vi "test_fpga_se_main.vi"() -> ()   [LabVIEW 2016]
uses:
  <vilib>/Platform/TimedLoop/XDataNode/timing_clust.ctl
  <vilib>/Platform/TimedLoop/XDataNode/nitl_modes.ctl
  <vilib>/Platform/TimedLoop/XDataNode/wakeup.ctl
  <vilib>/rvi/Emulation/niFpgaSctlEmulationGetInTimedLoop.vi
  <vilib>/rvi/Emulation/niFpgaEmulationReportErrorSimple.vi
  <vilib>/rvi/Emulation/niFpgaGetClockAttributes.vi
  <vilib>/rvi/Emulation/niFpgaCriticalErrorInLSC.vi
  <vilib>/Platform/TimedLoop/XDataNode/XDataNode.xnode
  <vilib>/Platform/TimedLoop/XDataNode/XDNodeRunTimeDep.lvlib
panel:
  out "debug":cluster{"blanking":u32, "pixelEvent":bool}
  out "se.o.position":T1 {"outputInt"."x" format="%.16g"; "outputInt"."y" format="%.16g"}
  out "blankingOff":bool
  in  "scanClocks":T2={"se.mot.p.clocks"={"moveToDecFactor"=0, "moveToWaveSize"=0, "se.mot.p.invDec"=0.0}, "se.p.clocks"={"outputRate"=0, "fastDecFactor"=0, "outWaveSizeFast"=0, "pplUpsampling"=0, "numLines"=0, "se.p.fastInvDec"=0.0, "se.p.slowUpStep"=0.0, "se.p.outWaveSizeSlow"=0, "blankingMax"=0, "se.p.fastBlanking"={"startFwd"=0, "endFwd"=0, "startBwd"=0, "endBwd"=0, "disableBlanking"=FALSE, "useCoarseCounter"=TRUE}}}
  out "indices":T3
  in  "outputParams":T4
  out "se.mot.s.running":bool
  out "outputNorm":T5
  out "clocksOut":T6
  in  "se.p.modes":T7
  in  "se.mot.p.target":cluster{"x":fxp<+/-,16,1>, "y":fxp<+/-,16,1>}
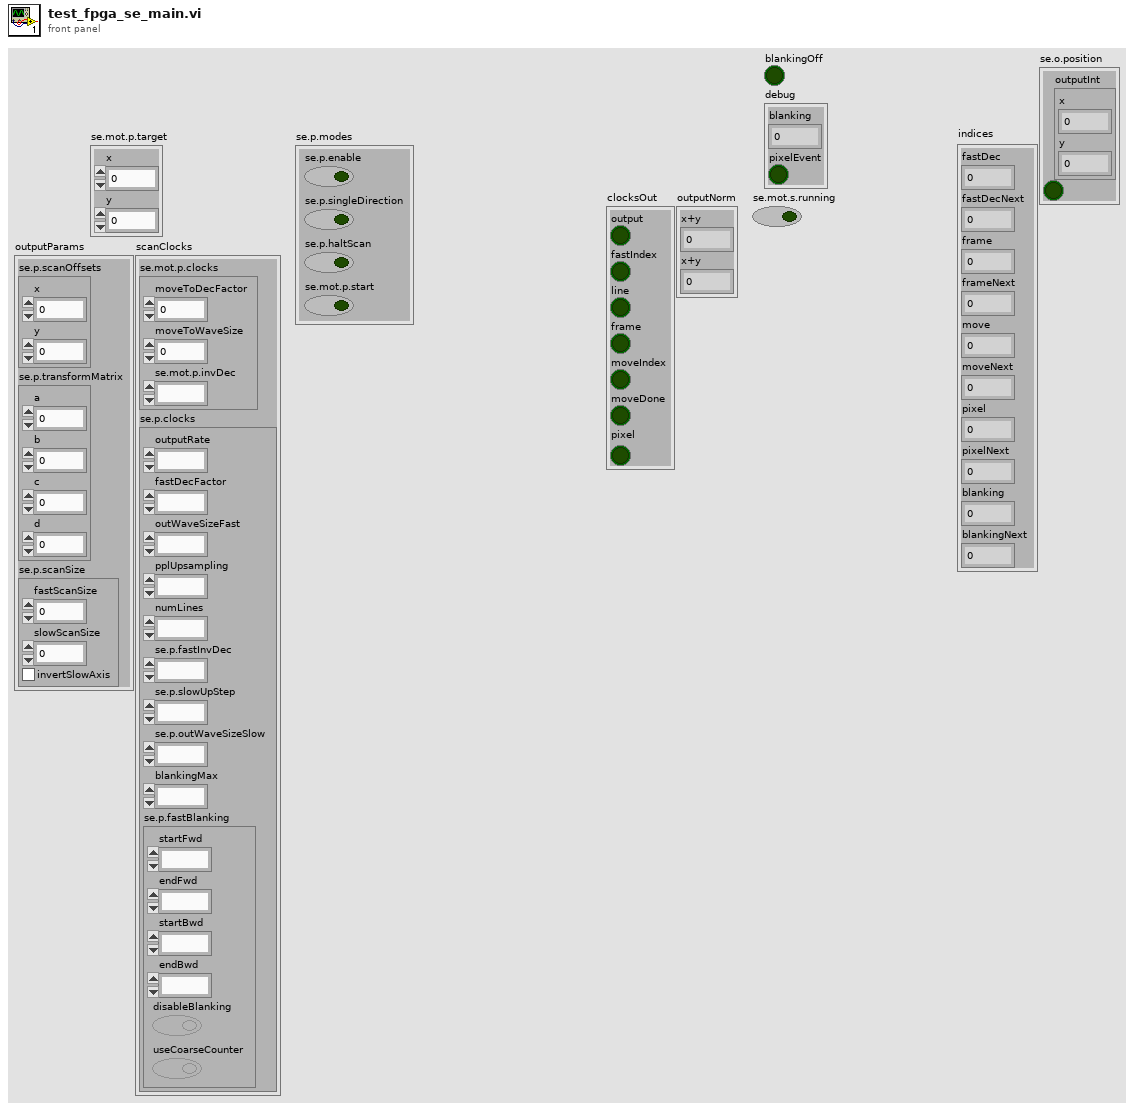
[diagram p1: front panel]
types:
  T1 = cluster{"outputInt":cluster{"y":fxp<+/-,16,1>, "y":fxp<+/-,16,1>}, bool}
  T2 = cluster{"se.mot.p.clocks":cluster{"moveToDecFactor":u16, "moveToWaveSize":u16, "se.mot.p.invDec":fxp<+,16,0>}, "se.p.clocks":cluster{"outputRate":u16, "fastDecFactor":u16, "outWaveSizeFast":u16, "pplUpsampling":u16, "numLines":u16, "se.p.fastInvDec":fxp<+,22,0>, "se.p.slowUpStep":fxp<+,28,0>, "se.p.outWaveSizeSlow":u16, "blankingMax":u32, "se.p.fastBlanking":cluster{"startFwd":u32, "endFwd":u32, "startBwd":u32, "endBwd":u32, "disableBlanking":bool, "useCoarseCounter":bool}}}
  T3 = cluster{"fastDec":u16, "fastDecNext":u16, "frame":u16, "frameNext":u16, "move":u16, "moveNext":u16, "pixel":u16, "pixelNext":u16, "blanking":u32, "blankingNext":u32}
  T4 = cluster{"se.p.scanOffsets":cluster{"x":fxp<+/-,16,1>, "y":fxp<+/-,16,1>}, "se.p.transformMatrix":cluster{"a":fxp<+/-,18,2>, "b":fxp<+/-,18,2>, "c":fxp<+/-,18,2>, "d":fxp<+/-,18,2>}, "se.p.scanSize":cluster{"fastScanSize":fxp<+,17,1>, "slowScanSize":fxp<+,17,1>, "invertSlowAxis":bool}}
  T5 = cluster{"x+y":fxp<+/-,18,2>, "x+y":fxp<+/-,18,2>}
  T6 = cluster{"output":bool, "fastIndex":bool, "line":bool, "frame":bool, "moveIndex":bool, "moveDone":bool, "pixel":bool}
  T7 = cluster{"se.p.enable":bool, "se.p.singleDirection":bool, "se.p.haltScan":bool, "se.mot.p.start":bool}
  T8 = typedef "XDNodeRunTimeDep.lvlib/timing_clust.ctl" = cluster{"Expected End [f-1]":u64, "Actual End [f-1]":u64, "Finished Late? [f-1]":bool, "Expected End [i-1]":u64, "Actual End [i-1]":u64, "Finished Late? [i-1]":bool, "Expected Start [i]":u64, "Actual Start [i]":u64, "Expected Start [f]":u64, "Actual Start [f]":u64, "Source Name":string, "Structure Name":string, "Period":i64, "Deadline":i64, "Offset":i64, "Start":i64, "Priority":i32, "Timeout":i32, "Mode":T9, "Wakeup Reason":T10, "Error":errorcluster, "Source Type":string, "Secondary Source Type":string, "Global End Time":u64, "Global Start Time":u64, "Frame Duration":u64, "Iteration Duration":u64, "Assigned CPU":i32, "I/O Scan Engine Mode":u32}
  T9 = typedef "XDNodeRunTimeDep.lvlib/nitl_modes.ctl" = enum32{"No Change", "Process missed periods, maintain original phase", "Discard missed periods, maintain original phase", "Process missed periods, ignore original phase", "Discard missed periods, ignore original phase"}
  T10 = typedef "XDNodeRunTimeDep.lvlib/wakeup.ctl" = enum32{"Normal", "Aborted", "Asynchronous wakeup", "Timing source error", "Timed loop error", "Timeout"}
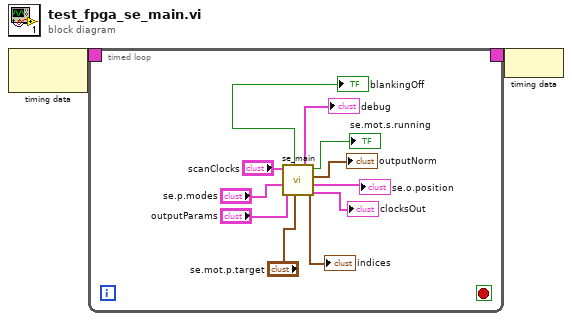
[diagram p0: block diagram]
diagram:
  n1 = node-c288() -> (w2:T8)  [unwired: 1 in]
  n2 = timed-loop {
    timing: w2 -> [_]
    timing-out: [_] -> w1
    stop <- _ stop-if-true
    n3 = call "se_main.vi"("se.mot.p.target"="se.mot.p.target", "outputParams"="outputParams", "se.p.modes"="se.p.modes", "scanClocks"="scanClocks") -> ("clocksOut"=→"clocksOut":T6, "se.o.position"=→"se.o.position":T1, "se.mot.s.origin"=→"outputNorm":T5, "se.mot.s.running"=→"se.mot.s.running":bool, "indices"=→"indices":T3, "debug"=→"debug":cluster{"blanking":u32, "pixelEvent":bool}, "blankingOff"=→"blankingOff":bool)  [unwired: 1 in]
  }
  n4 = node-c288(w1) -> ()
